vi "Meta Data to TDMS File.vi"(6 "Channel name":string, 7 "Group name":string, 8 "Error In":errorcluster, 9 "Name":string, 10 "Value":variant, 11 "File Path":path) -> (0 "Error Out":errorcluster, 3 "File Path out":path)   [LabVIEW 2016]
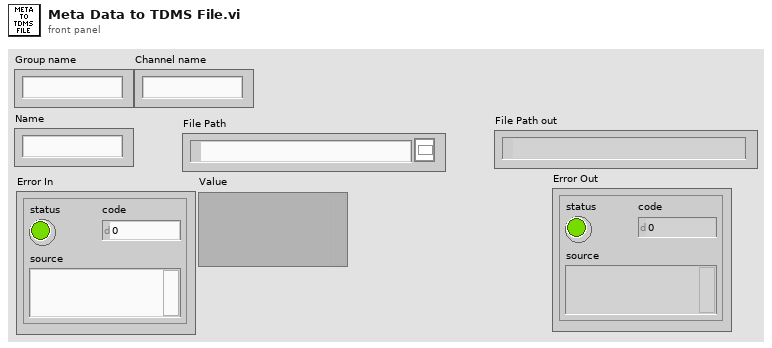
[diagram p1: front panel]
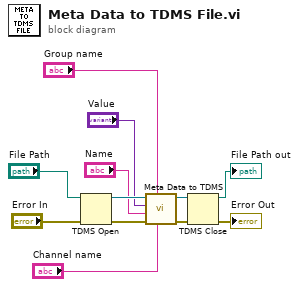
[diagram p0: block diagram]
diagram:
  n1 = TDMS Open(8:"Error In", 11:"File Path") -> (0:w5:errorcluster, 3:w11:refnum<k34>)  [unwired: 5 in]
  n2 = call "Meta Data to TDMS.vi"("Channel name"="Channel name", "Group name"="Group name", "Error In"=w5, "Name"="Name", "Value"="Value", "tdms file"=w11) -> ("Error Out"=w8:errorcluster, "tdms file out"=w10:refnum<k34>)  [unwired: 4 in]
  n3 = TDMS Close(8:w8, 11:w10) -> (0:→"Error Out":errorcluster, 3:→"File Path out":path)
